vi "Build Remaining Configuration.vi"(7 "Virtual Memory Unit in":refnum<class "Virtual Memory Unit.lvclass">, 8 "error in (no error)":errorcluster, 10 "Starting Address":u16 format="%04x", 11 "Message in":refnum<class "Message.lvclass">) -> (0 "error out":errorcluster, 2 "Next Available Address":u16 format="%04x", 3 "Message out":refnum<class "Message.lvclass">, 5 "Virtual Memory Unit out":refnum<class "Virtual Memory Unit.lvclass">)   [LabVIEW 2020, in "BCI-1553 API.lvlib" / "Message.lvclass"]
doc: "Fills the remaining memory locations in the control/status block with 0000. This is just to ensure that there is no other possible uninitialized content in those locations."
uses:
  Message.lvclass
  Dependencies/Virtual Memory Unit/Virtual Memory Unit.lvclass
  BCI-1553 API.lvlib
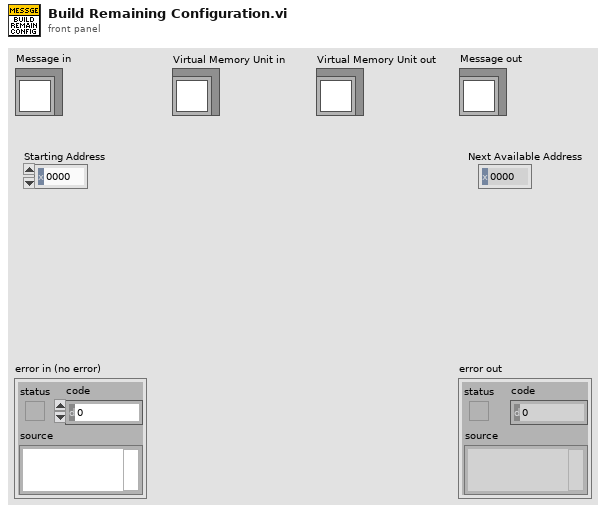
[diagram p1: front panel]
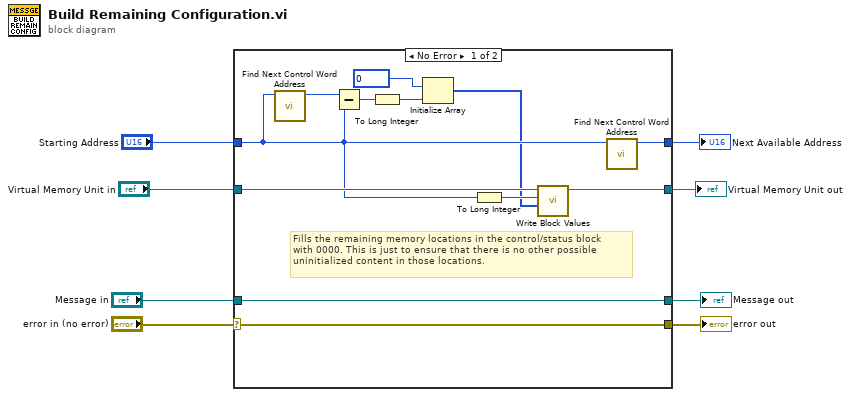
[diagram p0: block diagram]
diagram:
  n1 = case shown="No Error" "error in (no error)" {
    selector: "error in (no error)" -> [w19 w23]
    tunnel: [w19 w23] -> w7
    tunnel: [w20 w22] -> w5
    tunnel: "Message in" -> [w20 w22]
    tunnel: "Starting Address" -> [w10 w21]
    tunnel: [w14 w21] -> w3
    tunnel: "Virtual Memory Unit in" -> [w13 _]
    tunnel: [w12 _] -> w1
    frame No Error {
      # "Fills the remaining memory locations in the control/status block\nwith 0000. This is just to ensure that there is no other possible\nuninitialized content in those locations."
      n2 = call "Find Next Control Word Address.vi"("Starting Address"=w10) -> ("0xHHHX Address"=w15:u16)  [unwired: 10 in]
      n3 = Subtract(x=w15, y=w10) -> (x-y=w18:u16)
      n4 = To Long Integer(number=w18) -> (32bit integer=w17:i32)
      n5 = Initialize Array(u16 0 ("element"), w17) -> (w9:u16[])
      n6 = To Long Integer(number=w10) -> (32bit integer=w11:i32)
      n7 = call "Write Block Values.vi"("Write Block"=w9, "Start Index"=w11, "Virtual Memory Unit in"=w13) -> ("Virtual Memory Unit out"=w12:refnum<class "Virtual Memory Unit.lvclass">)  [unwired: 7 in, 1 out]
      n8 = call "Find Next Control Word Address.vi"("Starting Address"=w10) -> ("0xHHHX Address"=w14:u16)  [unwired: 10 in]
    }
    frame Error {
    }
  }
  "error out" <- w7
  "Message out" <- w5
  "Virtual Memory Unit out" <- w1
  "Next Available Address" <- w3
